vi "Test UI-Bus.vi"() -> ()   [LabVIEW 2021]
panel:
  out "Array":string[](array[string])
  in  "Numeric":dbl
  in  "Numeric":dbl
  out "Waveform Chart":dbl(graph)
  in  "Tab Control":enum32{"Page 1", "Page 2"}(tab)
  in  "Tab Control 2":enum32{"Page 1", "Page 2"}(tab)
  in  "Boolean":bool
  out "Waveform Chart 2":dbl(graph)
  in  "String":string
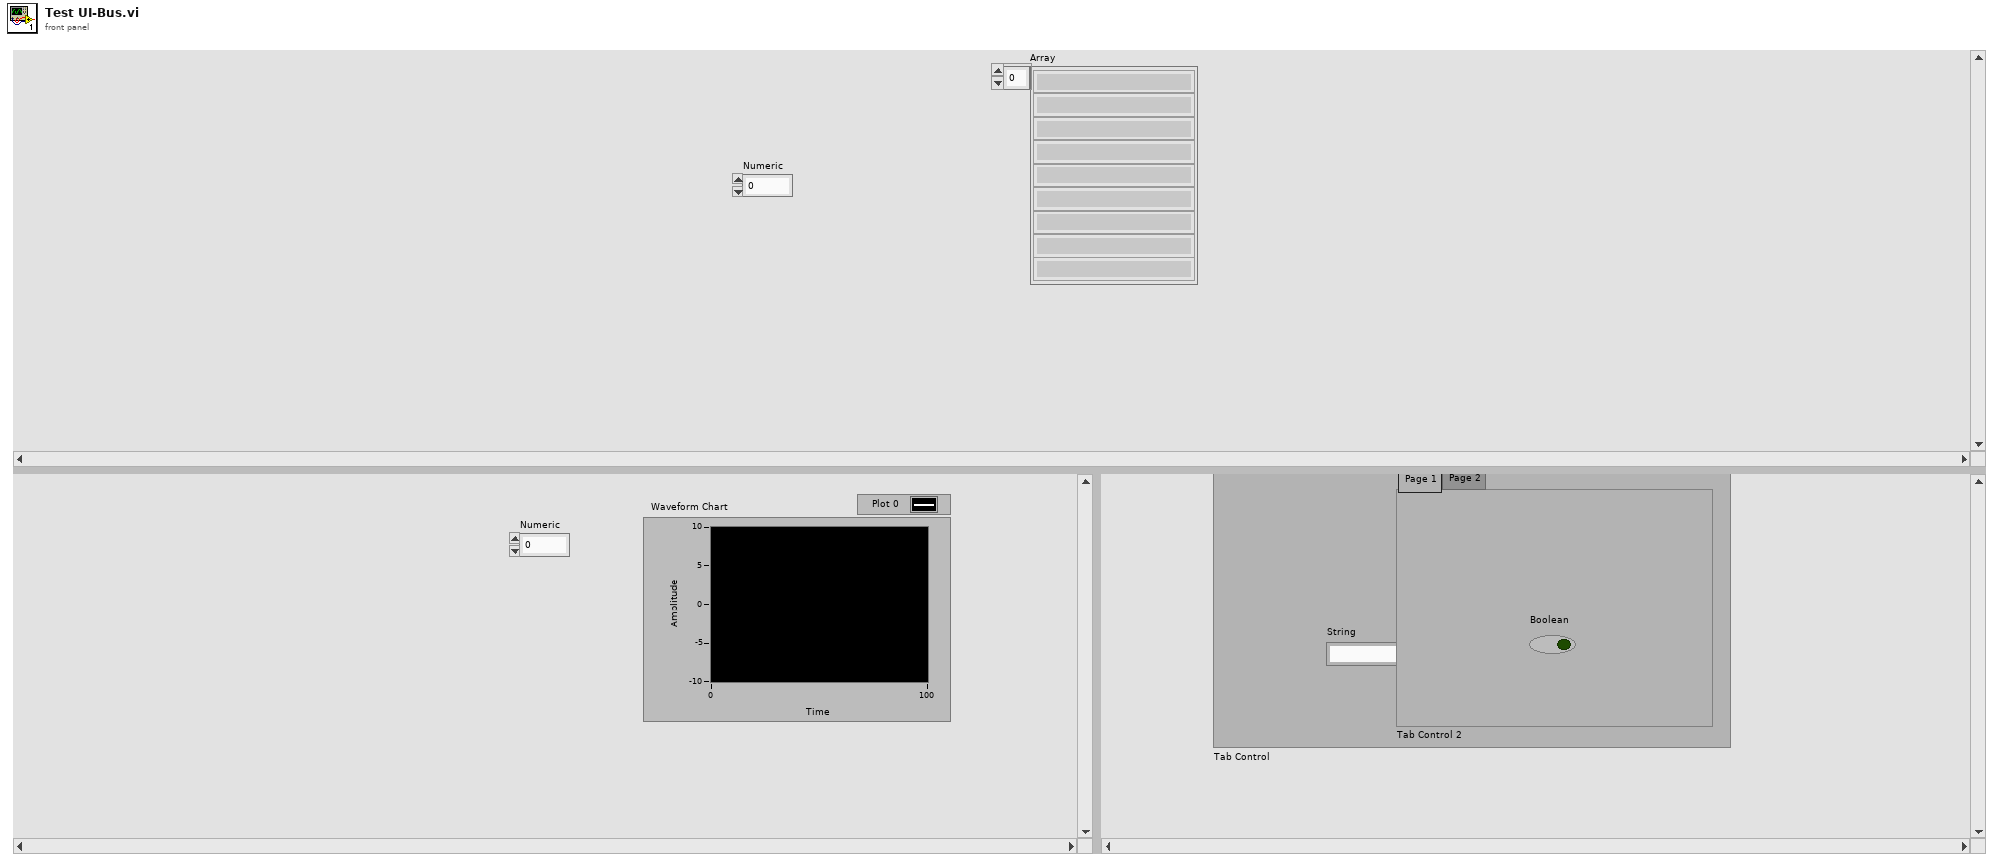
[diagram p1: front panel]
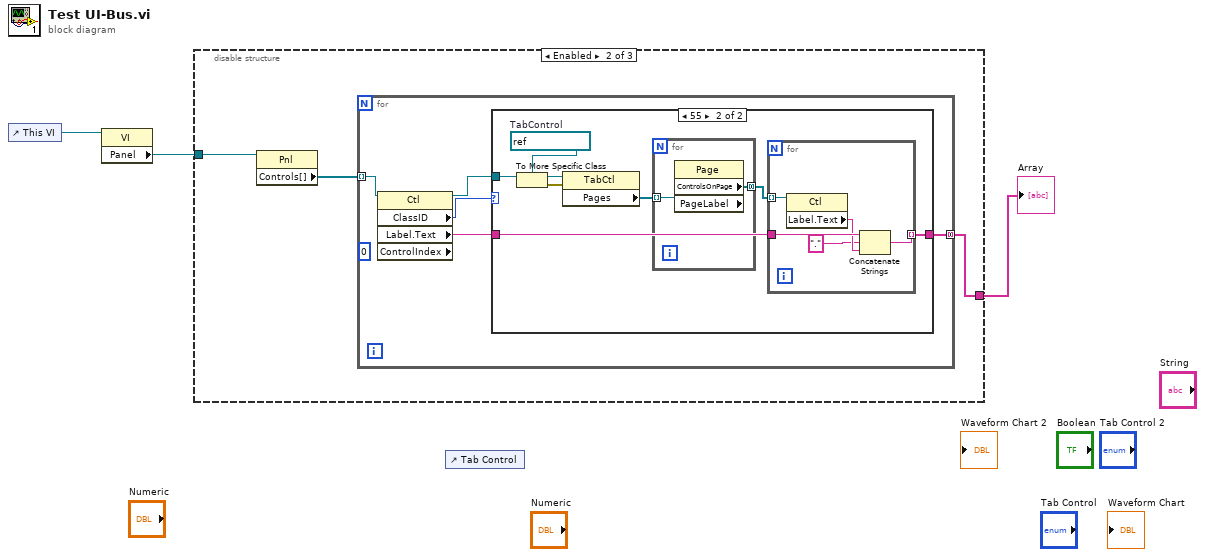
[diagram p0: block diagram]
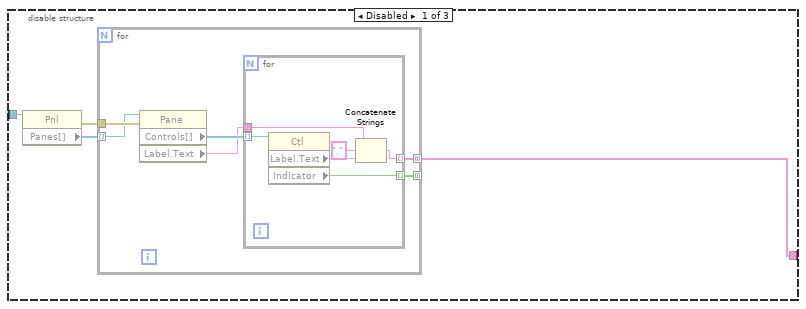
[diagram p2: hidden frame]
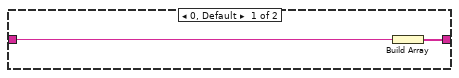
[diagram p3: hidden frame]
diagram:
  n1 = control-ref of="This VI"() -> (w3:refnum<vi>)
  n2 = property class="VI"(reference=w3) -> ("Panel"=w2:refnum<vi>)  [unwired: 1 in, 2 out]
  n3 = disable-structure shown="Enabled" {
    disable-tunnel: w2 -> [w6 w20 _]
    disable-tunnel: [w4 w22 _] -> w1
    frame Disabled {
      n4 = property class="Pnl"(reference=w6) -> (error out=w7:errorcluster, "Panes[]"=w5:refnum<vi>[])  [unwired: 1 in, 1 out]
      n5 = for {
        tunnel: w7 -> [w12]
        tunnel: w5 -> [w11] mode=indexing
        tunnel: [w10] -> w4 mode=concatenating
        tunnel: [w9] -> _ mode=concatenating
        n6 = property class="Pane"(reference=w11, error in=w12) -> ("Controls[]"=w13:refnum<vi>[], "Label.Text"=w8:string)  [unwired: 2 out]
        n7 = for {
          tunnel: w13 -> [w19] mode=indexing
          tunnel: [w16] -> w10 mode=indexing
          tunnel: [w17] -> w9 mode=indexing
          tunnel: w8 -> [w15]
          n8 = property class="Ctl"(reference=w19) -> ("Label.Text"=w18:string, "Indicator"=w17:bool)  [unwired: 1 in, 2 out]
          n9 = Concatenate Strings(w15, "." ("string"), w18) -> (w16:string)
        }
      }
    }
    frame Enabled {
      n10 = property class="Pnl"(reference=w20) -> ("Controls[]"=w21:refnum<vi>[])  [unwired: 1 in, 2 out]
      n11 = for {
        tunnel: w21 -> [w27] mode=indexing
        tunnel: [w23] -> w22 mode=concatenating
        (unwired) 0 ("Control Index")
        n12 = property class="Ctl" props=["ClassID", "Label", "Text", "ControlIndex"](reference=w27) -> (reference out=w25:refnum<vi>, "ClassID"=w26:u32, "Label.Text"=w24:string)  [unwired: 1 in, 2 out]
        n13 = case shown="55" w26 {
          tunnel: w25 -> [_ w37]
          tunnel: w24 -> [w29 w33]
          tunnel: [w28 w32] -> w23
          frame 0, Default {
            n14 = Build Array(w29) -> (w28:string[])
          }
          frame 55 {
            w36 = refnum<vi> refnum  # TabControl
            n15 = To More Specific Class(target class=w36, reference=w37) -> (specific class reference=w35:refnum<vi>, error out=w34:errorcluster)  [unwired: 1 in]
            n16 = property class="TabCtl"(reference=w35, error in=w34) -> ("Pages"=w31:refnum<vi>[])  [unwired: 2 out]
            n17 = for {
              tunnel: w31 -> [w39] mode=indexing
              tunnel: [w38] -> w30 mode=concatenating
              n18 = property class="Page" props=["ControlsOnPage", "PageLabel"](reference=w39) -> ("ControlsOnPage"=w38:refnum<vi>[])  [unwired: 1 in, 3 out]
            }
            n19 = for {
              tunnel: w30 -> [w42] mode=indexing
              tunnel: w33 -> [w43]
              tunnel: [w44] -> w32 mode=indexing
              n20 = property class="Ctl"(reference=w42) -> ("Label.Text"=w41:string)  [unwired: 1 in, 2 out]
              n21 = Concatenate Strings(w43, "." ("string"), w41) -> (w44:string)
            }
          }
        }
      }
    }
    frame Disabled {
    }
  }
  "Array" <- w1
  n22 = control-ref of="Tab Control"() -> ()  [unwired: 1 out]
